vi "Read Global Locked.vi"(7 "Semaphore Timeout":i32=-1, 8 "error in (no error)":errorcluster, 11 "Catapult in":refnum<class "Catapult.lvclass">) -> (0 "error out":errorcluster, 1 "Semaphore Timed Out":bool, 2 "Global":refnum<class "System.lvclass">, 3 "Catapult out":refnum<class "Catapult.lvclass">)   [LabVIEW 2013, in "Catapult.lvclass"]
uses:
  Catapult.lvclass
  System/System.lvclass
  Robot Global Data.vi
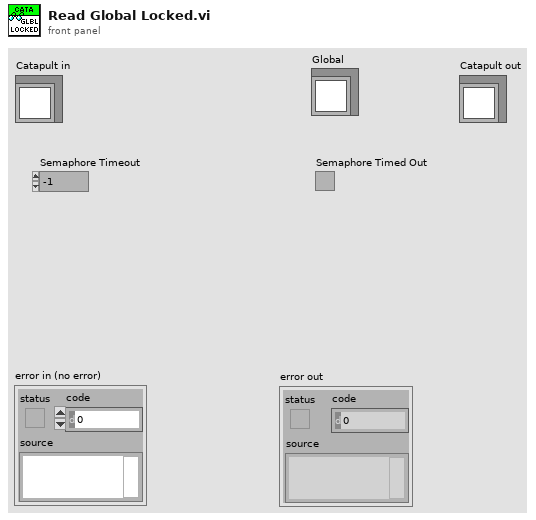
[diagram p1: front panel]
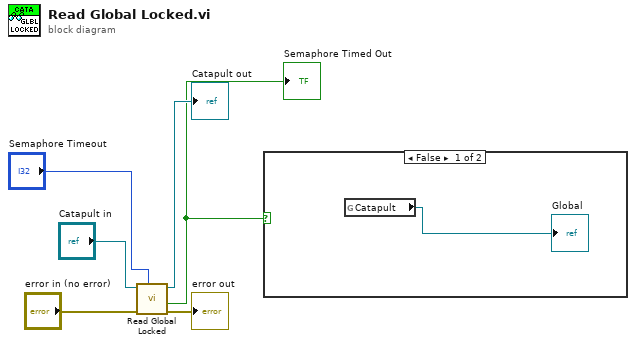
[diagram p0: block diagram]
diagram:
  n1 = call-parent "Read Global Locked.vi"("Semaphore Timeout"="Semaphore Timeout", "error in (no error)"="error in (no error)", "System in"="Catapult in") -> ("error out"=→"error out":errorcluster, "Semaphore Timed Out"=w1:bool, "System out"=→"Catapult out":refnum<class "Catapult.lvclass">)  [unwired: 5 in, 1 out]
  "Semaphore Timed Out" <- w1
  n2 = case shown="False" w1 {
    frame False {
      n3 = global read "Robot Global Data.vi" "Catapult"() -> (→"Global":refnum<class "Catapult.lvclass">)
    }
    frame True {
    }
  }
